vi "Select Manipulator Axis.vi"(9 "index":i32, 10 "Axis":bool[](array[boolean]), 11 "Num Axes":i32) -> (2 "Axis":bool[](array[boolean]))   [LabVIEW 2020, in "Dashboard.lvlib"]
uses:
  Dashboard.lvlib
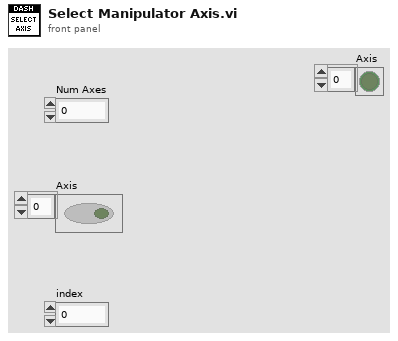
[diagram p1: front panel]
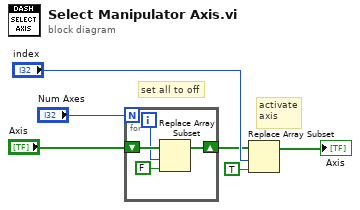
[diagram p0: block diagram]
diagram:
  # "set all to off"
  # "activate\naxis"
  n1 = for {
    N: "Num Axes" -> [_]
    shift-right: [w9] -> w4
    shift-left: "Axis" -> [w10]
    i -> [w8]
    n2 = Replace Array Subset(array=w10, new element=FALSE ("new element/subarray"), index=w8) -> (w9:bool[])
  }
  n3 = Replace Array Subset(array=w4, new element=TRUE ("new element/subarray"), index="index") -> (→"Axis":bool[])
